vi "UTILITY Convert String to TimeStamp.vi"(9 "Date":string) -> (1 "Resulting Date Stamp":timestamp format="%<%x>T", 2 "double precision float":dbl)   [LabVIEW 2016]
doc: "This VI convert a date/time string back to a time stamp."
uses:
  Type Definitions/UTILITY Date and Time.ctl
  <vilib>/Utility/miscctls.llb/LVDateTimeRec.ctl
panel:
  in  "date time rec":T1
  in  "date time rec 2":T2
  # "This control should have data in the form:\n4/30/2004"
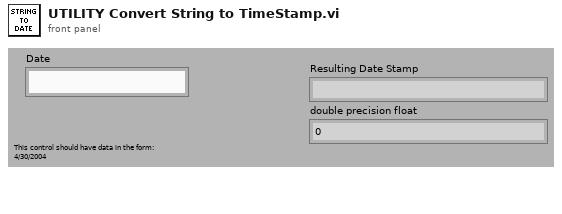
[diagram p1: front panel]
types:
  T1 = typedef "LVDateTimeRec.ctl" = cluster{"fractional second":dbl, "second":i32, "minute":i32, "hour":i32, "day of month":i32, "month":i32, "year":i32, "day of week":i32, "day of year":i32, "DST":i32}
  T2 = typedef "UTILITY Date and Time.ctl" = cluster{"second":i32, "minute":i32, "hour":i32, "day of month":i32, "month":i32, "year":i32, "day of week":i32, "day of year":i32, "is DST":i32, "fraction":dbl}
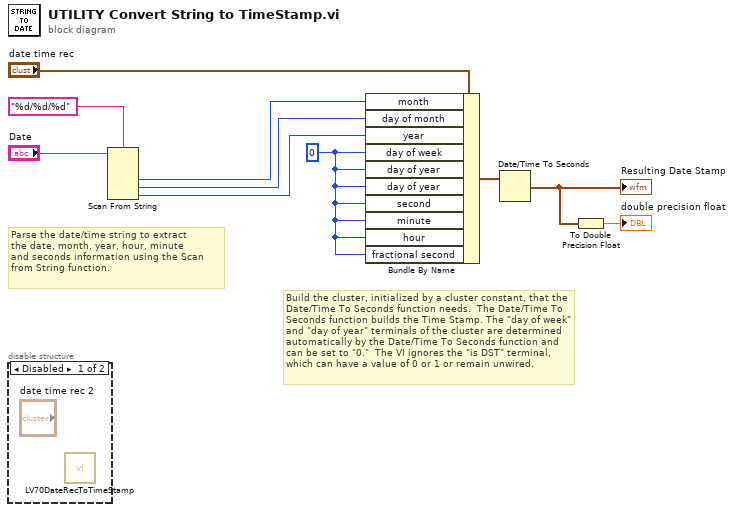
[diagram p0: block diagram]
diagram:
  w3 = 0
  # "Build the cluster, initialized by a cluster constant, that the Date/Time To Seconds function needs.  The Date/Time To Seconds function builds the Time Stamp. The \"day of week\" and \"day of year\" terminals of the cluster are determined automatically by the Date/Time To Seconds function and can be set to \"0.\"  The VI ignores the \"is DST\" terminal, which can have a value of 0 or 1 or remain unwired."
  # "Parse the date/time string to extract \nthe date, month, year, hour, minute \nand seconds information using the Scan\nfrom String function."
  n1 = disable-structure shown="Disabled" {
    frame Disabled {
      n2 = call "LV70DateRecToTimeStamp.vi"() -> ()  [unwired: 1 in, 1 out]
    }
    frame Enabled {
    }
  }
  n3 = Scan From String "Scan From String"(format string="%d/%d/%d", input string="Date") -> (output 1=w4:i32, output 2=w8:i32, output 3=w7:i32)  [unwired: 5 in, 3 out]
  n4 = Bundle By Name(cluster="date time rec", "month"=w4, "day of month"=w8, "year"=w7, "day of week"=w3, "day of year"=w3, "day of year"=w3, "second"=w3, "minute"=w3, "hour"=w3, "fractional second"=w3) -> (w5:T1)
  n5 = Date/Time To Seconds(2:w5) -> (0:w2:timestamp)  [unwired: 1 in]
  "Resulting Date Stamp" <- w2
  n6 = To Double Precision Float(number=w2) -> (double precision float=→"double precision float":dbl)
